vi "Set State.vi"(8 "error in (no error)":errorcluster, 10 "State":T1, 11 "Elevator Controller in":refnum<class "Elevator Controller.lvclass">) -> (0 "error out":errorcluster, 3 "Elevator Controller out":refnum<class "Elevator Controller.lvclass">)   [LabVIEW 2019, in "Elevator Controller.lvlib" / "Elevator Controller.lvclass"]
uses:
  Elevator Controller.lvclass
  State -Enum.ctl
  Elevator Controller.lvclass/Elevator Controller.ctl
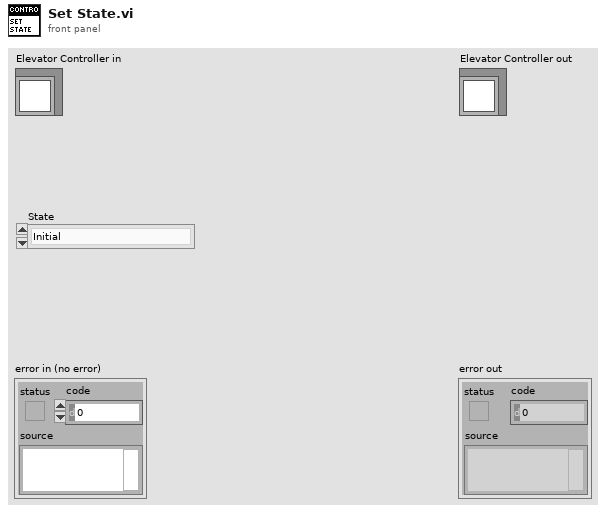
[diagram p1: front panel]
types:
  T1 = typedef "Elevator Controller.lvlib/Elevator Controller.lvclass/State -Enum.ctl" = enum16{"Initial", "Wait for First Request", "Start and Move", "Analysis", "Continue Travel", "Stop at Floor", "Open and Close Door Sequence", "No request Remaining", "Emergency Call", "Terminate Process"}
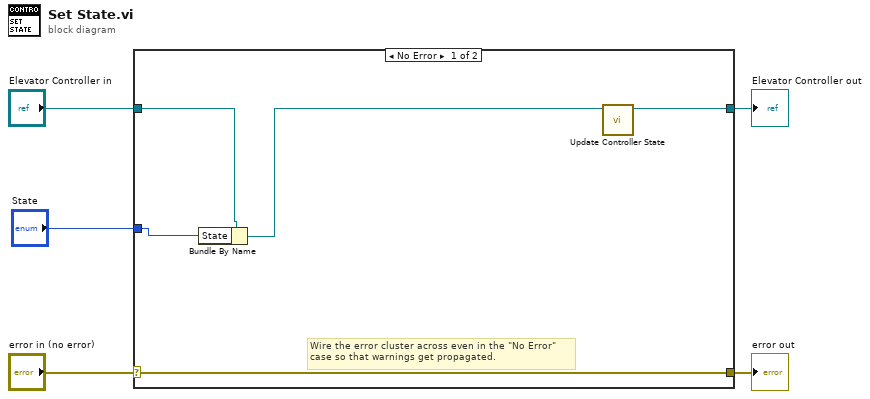
[diagram p0: block diagram]
diagram:
  n1 = case shown="No Error" "error in (no error)" {
    selector: "error in (no error)" -> [w10 w12]
    tunnel: [w10 w12] -> w4
    tunnel: [w7 w11] -> w2
    tunnel: "Elevator Controller in" -> [w8 w11]
    tunnel: "State" -> [w9 _]
    frame No Error {
      # "Wire the error cluster across even in the \"No Error\"\ncase so that warnings get propagated."
      n2 = Bundle By Name(cluster=w8, "State"=w9) -> (w6:refnum<class "Elevator Controller.lvclass">)
      n3 = call "Update Controller State.vi"("Elevator Controller in"=w6) -> ("Elevator Controller out"=w7:refnum<class "Elevator Controller.lvclass">)  [unwired: 9 in, 1 out]
    }
    frame Error {
    }
  }
  "error out" <- w4
  "Elevator Controller out" <- w2
